vi "subpanelHelper.vi"() -> ()   [LabVIEW 2013]
uses:
  M2AADTViews.lvlib
panel:
  in  "Apply exceptions?":bool
  out "error out":errorcluster
  in  "Exceptions":string[](array[string])
  in  "Make subpanels...":bool
  out "Subpanels":string[](array[string])
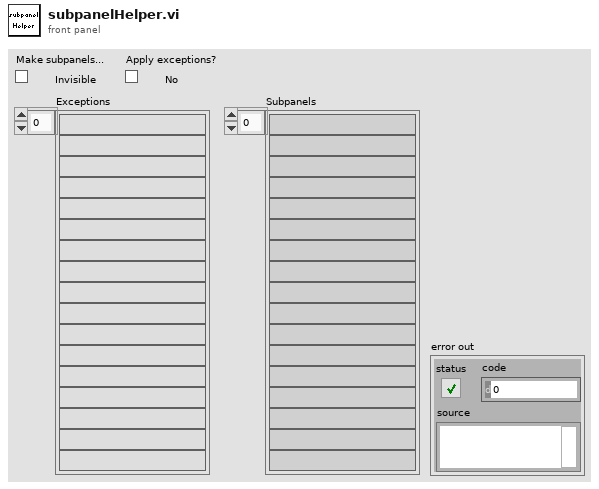
[diagram p1: front panel]
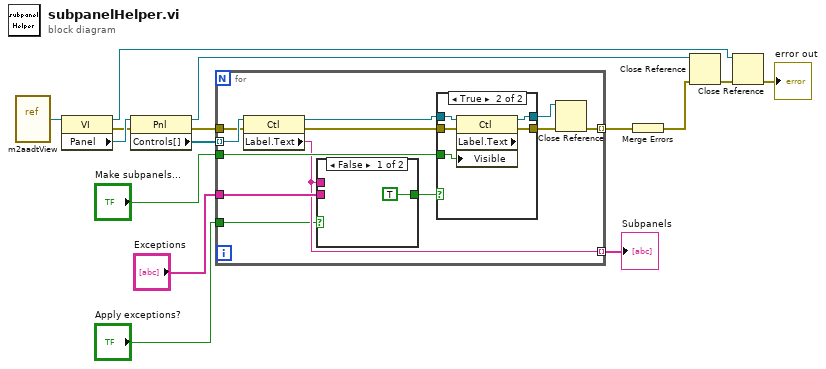
[diagram p0: block diagram]
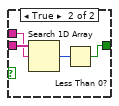
[diagram p2: hidden frame]
diagram:
  n1 = vi-ref "m2aadtView.vi"() -> (w15:refnum<vi>)
  n2 = property class="VI"(reference=w15) -> (reference out=w3:refnum<vi>, error out=w9:errorcluster, "Panel"=w14:refnum<vi>)  [unwired: 1 in]
  n3 = property class="Pnl"(reference=w14, error in=w9) -> (reference out=w4:refnum<vi>, error out=w8:errorcluster, "Controls[]"=w13:refnum<vi>[])
  n4 = for {
    tunnel: w13 -> [w27] mode=indexing
    tunnel: [w23] -> w12 mode=indexing
    tunnel: "Make subpanels..." -> [w25]
    tunnel: "Exceptions" -> [w24]
    tunnel: w8 -> [w21]
    tunnel: [w18] -> w7 mode=indexing
    tunnel: "Apply exceptions?" -> [w16]
    n5 = property class="Ctl"(reference=w27, error in=w21) -> (reference out=w26:refnum<vi>, error out=w20:errorcluster, "Label.Text"=w23:string)
    n6 = case shown="False" w16 {
      tunnel: w24 -> [_ w32]
      tunnel: w23 -> [_ w31]
      tunnel: [TRUE w29] -> w17
      frame False {
      }
      frame True {
        n7 = Search 1D Array(1D array=w32, element=w31) -> (index of element=w30:i32)  [unwired: 1 in]
        n8 = Less Than 0?(x=w30) -> (x < 0?=w29:bool)
      }
    }
    n9 = case shown="True" w17 {
      tunnel: w26 -> [w34 w39]
      tunnel: w25 -> [_ w38]
      tunnel: [w34 w37] -> w22
      tunnel: w20 -> [w33 w36]
      tunnel: [w33 w35] -> w19
      frame False {
      }
      frame True {
        n10 = property class="Ctl" props=["Label", "Text", "Visible"](reference=w39, error in=w36, "Visible"=w38) -> (reference out=w37:refnum<vi>, error out=w35:errorcluster)  [unwired: 1 out]
      }
    }
    n11 = Close Reference(reference=w22, error in (no error)=w19) -> (error out=w18:errorcluster)
  }
  "Subpanels" <- w12
  n12 = Merge Errors(w7) -> (w6:errorcluster)
  n13 = Close Reference(reference=w4, error in (no error)=w6) -> (error out=w5:errorcluster)
  n14 = Close Reference(reference=w3, error in (no error)=w5) -> (error out=→"error out":errorcluster)
